vi "XY Graph Sliced Mean & SDV Enter Data Dialog.vi"(7 "Input Message":string, 8 "Error In":errorcluster, 10 "X min":dbl, 11 "X max":dbl) -> (0 "Error Out":errorcluster, 3 "Slices Definition":T1={"Axis Start"=0.0, "Axis Stop"=0.0, "# Steps"=0, "Step Size"=1.0, "Step Definition"=enum."# Steps", "Upper Percentile"=1.0, "Lower Percentile"=1.0, "Min # Data Points/Slice"=1, "Output Abscissa Statistics Plots"=FALSE} {"Min # Data Points/Slice" min=0 max=100; "Lower Percentile" min=0.0 max=100.0; "Upper Percentile" min=0.0 max=100.0; "Step Size" min=1.0; "# Steps" min=1}, 4 "Cancelled?":bool)   [LabVIEW 2021, in "XY Graph Add-Ons.lvlib"]
uses:
  XY Graph Add-Ons.lvlib
  XY Graph Slides Mean & SDV Step Definition.ctl
panel:
  in  "Use Data Min/Max":bool
  in  "Slices Definition":T1={"Axis Start"=0.0, "Axis Stop"=0.0, "# Steps"=1, "Step Size"=1.0, "Step Definition"=enum."# Steps", "Upper Percentile"=100.0, "Lower Percentile"=0.0, "Min # Data Points/Slice"=1, "Output Abscissa Statistics Plots"=FALSE} {"Min # Data Points/Slice" min=0 max=100; "Lower Percentile" min=0.0 max=100.0; "Upper Percentile" min=0.0 max=100.0; "Step Size" min=0.0; "# Steps" min=1}
  out "Message":string="Enter the first (start) and last (stop) values to consider for the analysis, as well as the number of intervals (# Steps) in which to divide the range of values:"
  in  "Cancel":bool
  in  "OK":bool
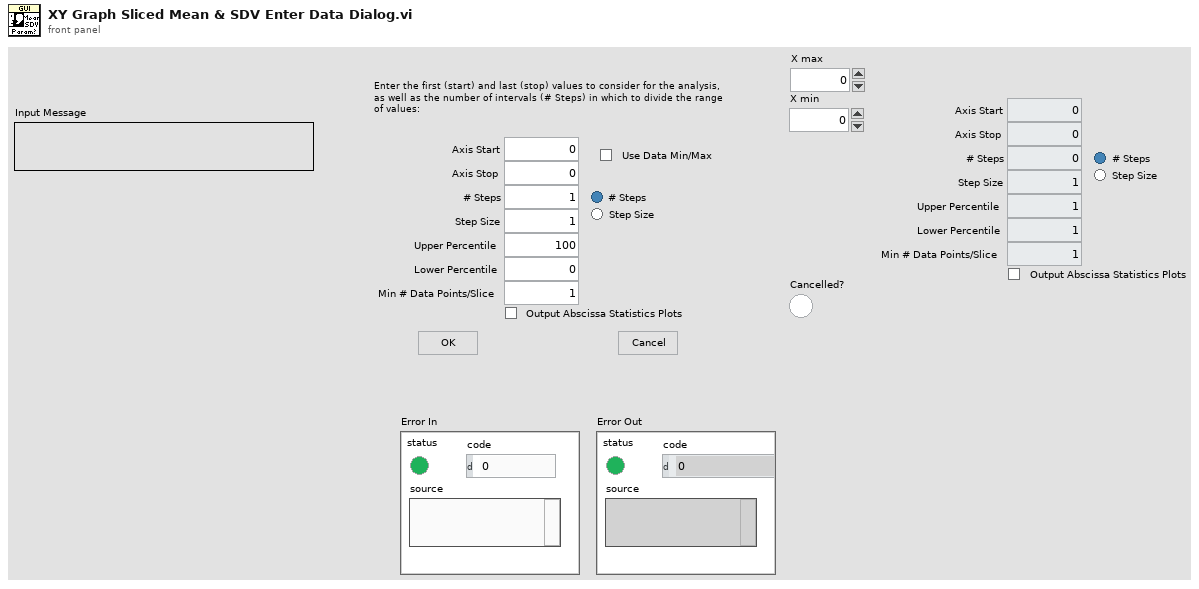
[diagram p1: front panel]
types:
  T1 = typedef "XY Graph Add-Ons.lvlib/XY Graph Slides Mean & SDV Step Definition.ctl" = cluster{"Axis Start":dbl, "Axis Stop":dbl, "# Steps":i32, "Step Size":dbl, "Step Definition":enum32{"# Steps", "Step Size"}, "Upper Percentile":dbl, "Lower Percentile":dbl, "Min # Data Points/Slice":i32, "Output Abscissa Statistics Plots":bool}
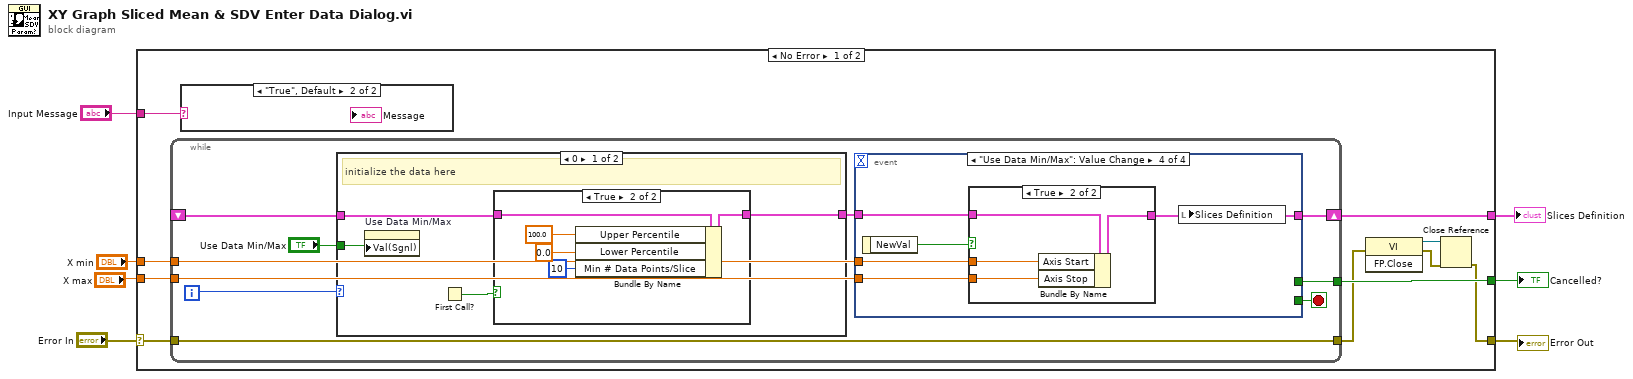
[diagram p0: block diagram]
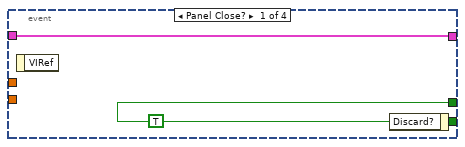
[diagram p5: hidden frame]
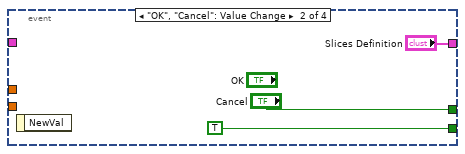
[diagram p6: hidden frame]
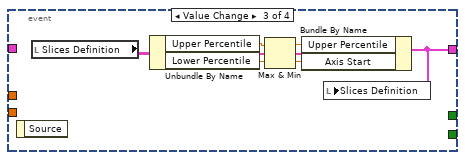
[diagram p7: hidden frame]
diagram:
  n1 = case shown="No Error" "Error In" {
    selector: "Error In" -> [w12 w60]
    tunnel: [w17 _] -> w7
    tunnel: [w16 _] -> w3
    tunnel: "Input Message" -> [w8 _]
    tunnel: [w13 w60] -> w4
    tunnel: "X min" -> [w10 _]
    tunnel: "X max" -> [w9 _]
    frame No Error {
      n2 = while {
        tunnel: [w26] -> w17
        shift-right: [w23] -> w16
        shift-left: _ -> [w24]
        tunnel: w12 -> [w21]
        tunnel: [w21] -> w11
        tunnel: w10 -> [w20]
        tunnel: w9 -> [w19]
        i -> [w25]
        stop <- w27 stop-if-true
        n3 = case shown="0" w25 {
          tunnel: w24 -> [w29 w38]
          tunnel: [w30 w38] -> w22
          tunnel: "Use Data Min/Max" -> [w28 _]
          frame 0 {
            # "initialize the data here"
            n4 = property on="Use Data Min/Max" class="Bool (strict)"("Val(Sgnl)"=w28) -> ()  [unwired: 2 in, 2 out]
            n5 = First Call?() -> (First Call?: T/F=w31:bool)
            n6 = case shown="True" w31 {
              tunnel: w29 -> [w32 w37]
              tunnel: [w32 w36] -> w30
              frame False {
              }
              frame True {
                n7 = Bundle By Name(cluster=w37, "Upper Percentile"=100.0, "Lower Percentile"=0.0, "Min # Data Points/Slice"=10) -> (w36:T1)
              }
            }
          }
          frame 1, Default {
          }
        }
        n8 = event shown="[3] \"Use Data Min/Max\": Value Change" {
          selector: _ -> [_ _ _ _]
          dyn-events: _ -> [_ _ _ _]
          timeout: _ -> [_ _ _ _]
          tunnel: [w40 TRUE ("Discard?") _ _] -> w27
          tunnel: [w40 "Cancel" _ _] -> w26
          tunnel: [w39 "Slices Definition" w44 w51] -> w23
          tunnel: w22 -> [w39 _ _ w54]
          tunnel: w20 -> [_ _ _ w53]
          tunnel: w19 -> [_ _ _ w52]
          event Panel Close? {
            w40 = TRUE ("Discard?")
            n9 = event-data() -> ()  [unwired: 1 in, 1 out]
            n10 = event-data("Discard?"=w40) -> ()  [unwired: 1 in, 1 out]
          }
          event "OK", "Cancel": Value Change {
            n11 = event-data() -> ()  [unwired: 1 in, 1 out]
          }
          event Value Change {
            n12 = event-data() -> ()  [unwired: 1 in, 1 out]
            n13 = local read "Slices Definition"() -> (w47:T1)
            n14 = Unbundle By Name(w47) -> ("Upper Percentile"=w49:dbl, "Lower Percentile"=w48:dbl)
            n15 = Max & Min(x=w49, y=w48) -> (max(x,y)=w46:dbl, min(x,y)=w45:dbl)
            n16 = Bundle By Name(cluster=w47, "Upper Percentile"=w46, "Axis Start"=w45) -> (w44:T1)
            n17 = local write "Slices Definition"(w44) -> ()
          }
          event "Use Data Min/Max": Value Change {
            n18 = event-data() -> ("NewVal"=w50:bool)  [unwired: 1 in]
            n19 = case shown="True" w50 {
              tunnel: w54 -> [w55 w59]
              tunnel: w53 -> [_ w58]
              tunnel: w52 -> [_ w57]
              tunnel: [w55 w56] -> w51
              frame False {
              }
              frame True {
                n20 = Bundle By Name(cluster=w59, "Axis Start"=w58, "Axis Stop"=w57) -> (w56:T1)
              }
            }
            n21 = local write "Slices Definition"(w51) -> ()
          }
        }
      }
      n22 = case shown="\"True\", Default" w8 {
        frame "" {
        }
        frame "True", Default {
        }
      }
      n23 = invoke class="VI" method="FP.Close"(error in=w11) -> (reference out=w15:refnum<vi>, error out=w14:errorcluster)  [unwired: 2 in, 1 out]
      n24 = Close Reference(reference=w15, error in (no error)=w14) -> (error out=w13:errorcluster)
    }
    frame Error {
    }
  }
  "Cancelled?" <- w7
  "Error Out" <- w4
  "Slices Definition" <- w3
